vi "CMN_Arr2Str_2.vi"(9 "separator":string, 10 "Array in":string[](array[string])) -> (2 "string out":string)   [LabVIEW 2016]
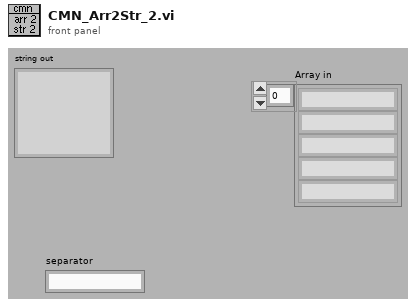
[diagram p1: front panel]
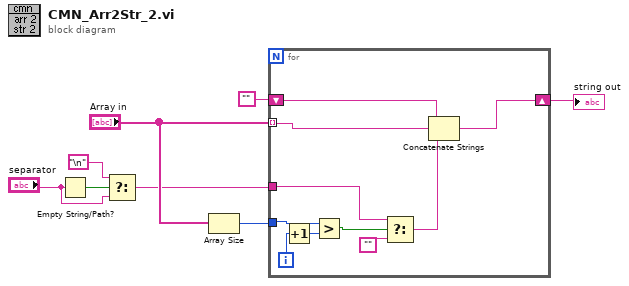
[diagram p0: block diagram]
diagram:
  n1 = Empty String/Path?(string/path="separator") -> (empty?=w4:bool)
  n2 = Select(t="\n", s=w4, f="separator") -> (s? t:f=w1:string)
  n3 = Array Size(array="Array in") -> (size(s)=w5:i32)
  n4 = for {
    tunnel: "Array in" -> [w16] mode=indexing
    shift-right: [w18] -> w7
    shift-left: "" -> [w17]
    tunnel: w5 -> [w15]
    tunnel: w1 -> [w9]
    i -> [w14]
    n5 = Increment(x=w14) -> (x+1=w10:i32)
    n6 = Greater?(x=w15, y=w10) -> (0:w13:bool)
    n7 = Select(t=w9, s=w13, f="") -> (s? t:f=w11:string)
    n8 = Concatenate Strings(w17, w16, w11) -> (w18:string)
  }
  "string out" <- w7
